vi "test-transform2d.vi"() -> ()   [LabVIEW 2019]
uses:
  <vilib>/Rock Robotics/WPI/ThirdParty/JAS_Junk/TrajLib/Translation_Equals.vi
  <vilib>/Rock Robotics/WPI/ThirdParty/JAS_Junk/TrajLib/Rotation_Equals.vi
  <vilib>/Rock Robotics/WPI/ThirdParty/JAS_Junk/TrajLib/Transform_Create_PosePose.vi
  <vilib>/Rock Robotics/WPI/ThirdParty/JAS_Junk/TrajLib/Pose_TransformBy.vi
  <vilib>/Rock Robotics/WPI/ThirdParty/JAS_Junk/TrajLib/Util_CalcDist.vi
  <vilib>/Rock Robotics/WPI/ThirdParty/JAS_Junk/TrajLib/Rotation_UnaryMinus.vi
  <vilib>/Rock Robotics/WPI/ThirdParty/JAS_Junk/TrajLib/Translation_RotateBy.vi
  <vilib>/Rock Robotics/WPI/ThirdParty/JAS_Junk/TrajLib/Translation_Minus.vi
  <vilib>/Rock Robotics/WPI/ThirdParty/JAS_Junk/TrajLib/Rotation_Minus.vi
  <vilib>/Rock Robotics/WPI/ThirdParty/JAS_Junk/TrajLib/Translation_Plus.vi
  <vilib>/Rock Robotics/WPI/ThirdParty/JAS_Junk/TrajLib/Rotation_Plus.vi
  <vilib>/Rock Robotics/WPI/ThirdParty/JAS_Junk/TrajLib/Rotation_RotateBy.vi
  <vilib>/Rock Robotics/WPI/ThirdParty/JAS_Junk/TrajLib/Rotation_CreateXY.vi
  <vilib>/Rock Robotics/WPI/ThirdParty/JAS_Junk/TrajLib/Trajectory_Library.lvlib
panel:
  out "T5 - ANG = 43 Deg":dbl
  out "T5 - Y2 = 4.4":dbl
  out "T5 - X2= -3.33":dbl
  out "T5 - Y = 4.4":dbl
  out "T5 - X = -3.33":dbl
  out "T4 -- Deg -- 0":dbl
  out "T4 -- y -- 0":dbl
  out "T4 -- X -- 0":dbl
  out "T3 - False":bool
  out "T2 - True":bool
  out "T1 -- Deg -- 0":dbl
  out "T1 -- y -- 0":dbl
  out "T1 -- X -- 0":dbl
  out "T0 -- Deg -- 0":dbl
  out "T0 -- y -- 0":dbl
  out "T0 -- X -- 0":dbl
  # "Transform2D Test  --- NOT DONE"
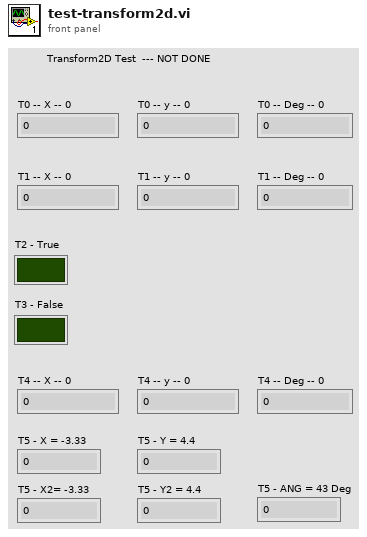
[diagram p1: front panel]
types:
  T1 = typedef "Trajectory_Library.lvlib/TRANSLATION2D.ctl" = cluster{"X":dbl, "Y":dbl}
  T2 = typedef "Trajectory_Library.lvlib/ROTATION2D.ctl" = cluster{"VALUE":dbl, "COS":dbl, "SIN":dbl}
  T3 = typedef "Trajectory_Library.lvlib/POSE2D.ctl" = cluster{"TRANSLATION":T1, "ROTATION":T2}
  T4 = typedef "Trajectory_Library.lvlib/TRANSFORM2D.ctl" = cluster{"TRANSLATION":T1, "ROTATION":T2}
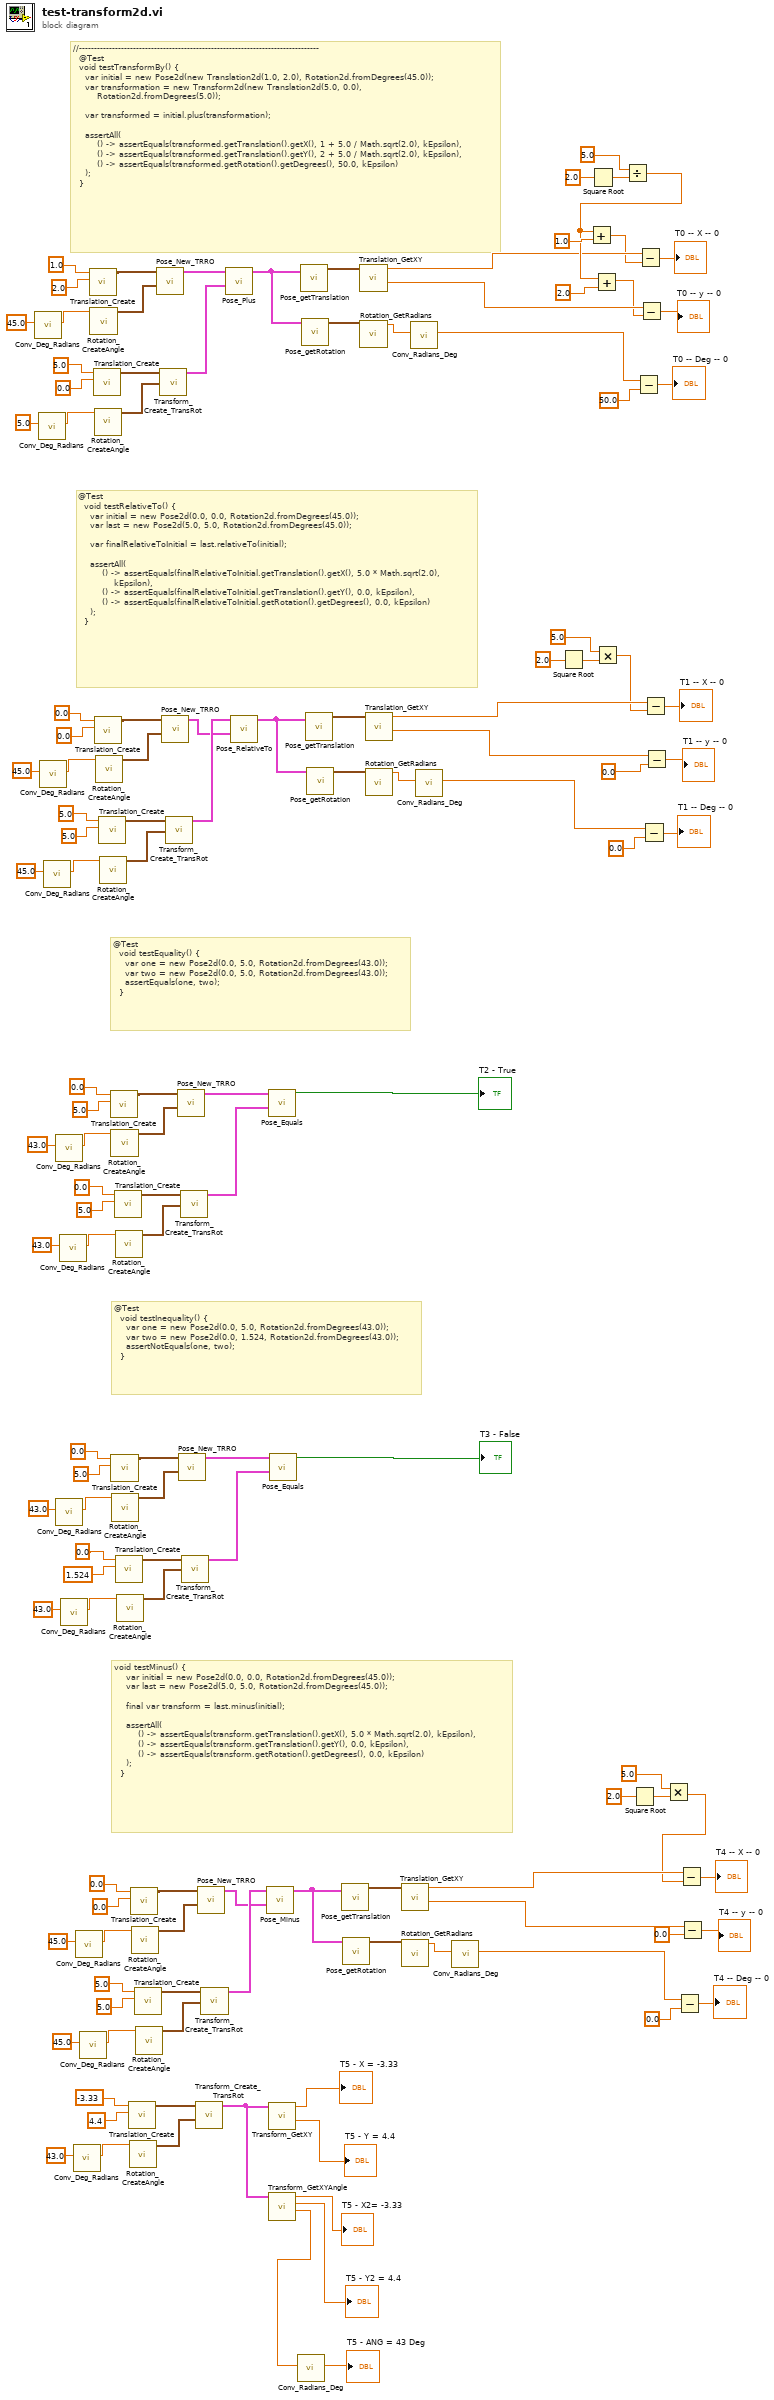
[diagram p0: block diagram]
diagram:
  # "void testMinus() {\n    var initial = new Pose2d(0.0, 0.0, Rotation2d.fromDegrees(45.0));\n    var last = new Pose2d(5.0, 5.0, Rotation2d.fromDegrees(45.0));\n\n    final var transform = last.minus(initial);\n\n    assertAll(\n        () -> assertEquals(transform.getTranslation().getX(), 5.0 * Math.sqrt(2.0), kEpsilon),\n        () -> assertEquals(transform.getTranslation().getY(), 0.0, kEpsilon),\n        () -> assertEquals(transform.getRotation().getDegrees(), 0.0, kEpsilon)\n    );\n  }"
  # "@Test\n  void testInequality() {\n    var one = new Pose2d(0.0, 5.0, Rotation2d.fromDegrees(43.0));\n    var two = new Pose2d(0.0, 1.524, Rotation2d.fromDegrees(43.0));\n    assertNotEquals(one, two);\n  }"
  # "@Test\n  void testEquality() {\n    var one = new Pose2d(0.0, 5.0, Rotation2d.fromDegrees(43.0));\n    var two = new Pose2d(0.0, 5.0, Rotation2d.fromDegrees(43.0));\n    assertEquals(one, two);\n  }"
  # "@Test\n  void testRelativeTo() {\n    var initial = new Pose2d(0.0, 0.0, Rotation2d.fromDegrees(45.0));\n    var last = new Pose2d(5.0, 5.0, Rotation2d.fromDegrees(45.0));\n\n    var finalRelativeToInitial = last.relativeTo(initial);\n\n    assertAll(\n        () -> assertEquals(finalRelativeToInitial.getTranslation().getX(), 5.0 * Math.sqrt(2.0),\n            kEpsilon),\n        () -> assertEquals(finalRelativeToInitial.getTranslation().getY(), 0.0, kEpsilon),\n        () -> assertEquals(finalRelativeToInitial.getRotation().getDegrees(), 0.0, kEpsilon)\n    );\n  }"
  # "//--------------------------------------------------------------------------------\n  @Test\n  void testTransformBy() {\n    var initial = new Pose2d(new Translation2d(1.0, 2.0), Rotation2d.fromDegrees(45.0));\n    var transformation = new Transform2d(new Translation2d(5.0, 0.0),\n        Rotation2d.fromDegrees(5.0));\n\n    var transformed = initial.plus(transformation);\n\n    assertAll(\n        () -> assertEquals(transformed.getTranslation().getX(), 1 + 5.0 / Math.sqrt(2.0), kEpsilon),\n        () -> assertEquals(transformed.getTranslation().getY(), 2 + 5.0 / Math.sqrt(2.0), kEpsilon),\n        () -> assertEquals(transformed.getRotation().getDegrees(), 50.0, kEpsilon)\n    );\n  }"
  n1 = call <vilib>:"Conv_Deg_Radians.vi"("Degress"=45.0) -> ("Radians"=w131:dbl)  [unwired: 10 in]
  n2 = call <vilib>:"Conv_Deg_Radians.vi"("Degress"=5.0) -> ("Radians"=w126:dbl)  [unwired: 10 in]
  n3 = call <vilib>:"Conv_Deg_Radians.vi"("Degress"=45.0) -> ("Radians"=w98:dbl)  [unwired: 10 in]
  n4 = call <vilib>:"Conv_Deg_Radians.vi"("Degress"=45.0) -> ("Radians"=w93:dbl)  [unwired: 10 in]
  n5 = call <vilib>:"Conv_Deg_Radians.vi"("Degress"=43.0) -> ("Radians"=w70:dbl)  [unwired: 10 in]
  n6 = call <vilib>:"Conv_Deg_Radians.vi"("Degress"=43.0) -> ("Radians"=w55:dbl)  [unwired: 10 in]
  n7 = call <vilib>:"Conv_Deg_Radians.vi"("Degress"=43.0) -> ("Radians"=w65:dbl)  [unwired: 10 in]
  n8 = call <vilib>:"Conv_Deg_Radians.vi"("Degress"=43.0) -> ("Radians"=w50:dbl)  [unwired: 10 in]
  n9 = call <vilib>:"Conv_Deg_Radians.vi"("Degress"=43.0) -> ("Radians"=w10:dbl)  [unwired: 10 in]
  n10 = call <vilib>:"Conv_Deg_Radians.vi"("Degress"=45.0) -> ("Radians"=w38:dbl)  [unwired: 10 in]
  n11 = call <vilib>:"Conv_Deg_Radians.vi"("Degress"=45.0) -> ("Radians"=w33:dbl)  [unwired: 10 in]
  n12 = call <vilib>:"Translation_Create.vi"("Y"=2.0, "X"=1.0) -> ("TRANSLATION"=w130:T1)  [unwired: 9 in]
  n13 = call <vilib>:"Rotation_CreateAngle.vi"("Angle"=w131) -> ("ROTATION"=w129:T2)  [unwired: 10 in]
  n14 = call <vilib>:"Translation_Create.vi"("Y"=0.0, "X"=5.0) -> ("TRANSLATION"=w124:T1)  [unwired: 9 in]
  n15 = call <vilib>:"Rotation_CreateAngle.vi"("Angle"=w126) -> ("ROTATION"=w123:T2)  [unwired: 10 in]
  n16 = call <vilib>:"Translation_Create.vi"("Y"=0.0, "X"=0.0) -> ("TRANSLATION"=w97:T1)  [unwired: 9 in]
  n17 = call <vilib>:"Rotation_CreateAngle.vi"("Angle"=w98) -> ("ROTATION"=w96:T2)  [unwired: 10 in]
  n18 = call <vilib>:"Translation_Create.vi"("Y"=5.0, "X"=5.0) -> ("TRANSLATION"=w91:T1)  [unwired: 9 in]
  n19 = call <vilib>:"Rotation_CreateAngle.vi"("Angle"=w93) -> ("ROTATION"=w90:T2)  [unwired: 10 in]
  n20 = call <vilib>:"Translation_Create.vi"("Y"=5.0, "X"=0.0) -> ("TRANSLATION"=w69:T1)  [unwired: 9 in]
  n21 = call <vilib>:"Rotation_CreateAngle.vi"("Angle"=w70) -> ("ROTATION"=w68:T2)  [unwired: 10 in]
  n22 = call <vilib>:"Translation_Create.vi"("Y"=5.0, "X"=0.0) -> ("TRANSLATION"=w54:T1)  [unwired: 9 in]
  n23 = call <vilib>:"Rotation_CreateAngle.vi"("Angle"=w55) -> ("ROTATION"=w53:T2)  [unwired: 10 in]
  n24 = call <vilib>:"Translation_Create.vi"("Y"=5.0, "X"=0.0) -> ("TRANSLATION"=w63:T1)  [unwired: 9 in]
  n25 = call <vilib>:"Rotation_CreateAngle.vi"("Angle"=w65) -> ("ROTATION"=w62:T2)  [unwired: 10 in]
  n26 = call <vilib>:"Translation_Create.vi"("Y"=1.524, "X"=0.0) -> ("TRANSLATION"=w48:T1)  [unwired: 9 in]
  n27 = call <vilib>:"Rotation_CreateAngle.vi"("Angle"=w50) -> ("ROTATION"=w47:T2)  [unwired: 10 in]
  n28 = call <vilib>:"Translation_Create.vi"("Y"=4.4, "X"=-3.33) -> ("TRANSLATION"=w9:T1)  [unwired: 9 in]
  n29 = call <vilib>:"Rotation_CreateAngle.vi"("Angle"=w10) -> ("ROTATION"=w8:T2)  [unwired: 10 in]
  n30 = call <vilib>:"Translation_Create.vi"("Y"=0.0, "X"=0.0) -> ("TRANSLATION"=w37:T1)  [unwired: 9 in]
  n31 = call <vilib>:"Rotation_CreateAngle.vi"("Angle"=w38) -> ("ROTATION"=w36:T2)  [unwired: 10 in]
  n32 = call <vilib>:"Translation_Create.vi"("Y"=5.0, "X"=5.0) -> ("TRANSLATION"=w31:T1)  [unwired: 9 in]
  n33 = call <vilib>:"Rotation_CreateAngle.vi"("Angle"=w33) -> ("ROTATION"=w30:T2)  [unwired: 10 in]
  n34 = call <vilib>:"Pose_New_TRRO.vi"("ROTATION"=w129, "TRANSLATION"=w130) -> ("outPOSE"=w122:T3)  [unwired: 9 in]
  n35 = call <vilib>:"Transform_Create_TransRot.vi"("ROTATION"=w123, "TRANSLATION"=w124) -> ("TRANSFORM"=w121:T4)  [unwired: 9 in]
  n36 = call <vilib>:"Pose_New_TRRO.vi"("ROTATION"=w96, "TRANSLATION"=w97) -> ("outPOSE"=w75:T3)  [unwired: 9 in]
  n37 = call <vilib>:"Transform_Create_TransRot.vi"("ROTATION"=w90, "TRANSLATION"=w91) -> ("TRANSFORM"=w76:T4)  [unwired: 9 in]
  n38 = call <vilib>:"Pose_New_TRRO.vi"("ROTATION"=w68, "TRANSLATION"=w69) -> ("outPOSE"=w61:T3)  [unwired: 9 in]
  n39 = call <vilib>:"Pose_New_TRRO.vi"("ROTATION"=w53, "TRANSLATION"=w54) -> ("outPOSE"=w46:T3)  [unwired: 9 in]
  n40 = call <vilib>:"Transform_Create_TransRot.vi"("ROTATION"=w62, "TRANSLATION"=w63) -> ("TRANSFORM"=w60:T4)  [unwired: 9 in]
  n41 = call <vilib>:"Transform_Create_TransRot.vi"("ROTATION"=w47, "TRANSLATION"=w48) -> ("TRANSFORM"=w45:T4)  [unwired: 9 in]
  n42 = call <vilib>:"Transform_Create_TransRot.vi"("ROTATION"=w8, "TRANSLATION"=w9) -> ("TRANSFORM"=w5:T4)  [unwired: 9 in]
  n43 = call <vilib>:"Pose_New_TRRO.vi"("ROTATION"=w36, "TRANSLATION"=w37) -> ("outPOSE"=w16:T3)  [unwired: 9 in]
  n44 = call <vilib>:"Transform_Create_TransRot.vi"("ROTATION"=w30, "TRANSLATION"=w31) -> ("TRANSFORM"=w17:T4)  [unwired: 9 in]
  n45 = call <vilib>:"Pose_Plus.vi"("other TRANSFORM"=w121, "in POSE"=w122) -> ("out POSE"=w119:T3)  [unwired: 9 in]
  n46 = call <vilib>:"Pose_RelativeTo.vi"("other POSE"=w75, "in POSE"=w76) -> ("out POSE"=w88:T3)  [unwired: 9 in]
  n47 = call <vilib>:"Pose_Minus.vi"("other TRANSFORM"=w16, "in POSE"=w17) -> ("outTRANSFORM"=w28:T4)  [unwired: 9 in]
  n48 = call <vilib>:"Pose_Equals.vi"("other POSE"=w60, "in POSE"=w61) -> ("Equals"=→"T2 - True":bool)  [unwired: 9 in]
  n49 = call <vilib>:"Transform_GetXY.vi"("inTRANSFORM"=w5) -> ("Y"=→"T5 - Y = 4.4":dbl, "X"=→"T5 - X = -3.33":dbl)  [unwired: 9 in]
  n50 = call <vilib>:"Transform_GetXYAngle.vi"("inTRANSFORM"=w5) -> ("Angle"=w1:dbl, "Y"=→"T5 - Y2 = 4.4":dbl, "X"=→"T5 - X2= -3.33":dbl)  [unwired: 8 in]
  n51 = call <vilib>:"Pose_Equals.vi"("other POSE"=w45, "in POSE"=w46) -> ("Equals"=→"T3 - False":bool)  [unwired: 9 in]
  n52 = call <vilib>:"Conv_Radians_Deg.vi"("Radians"=w1) -> ("Degrees"=→"T5 - ANG = 43 Deg":dbl)  [unwired: 10 in]
  n53 = call <vilib>:"Pose_getTranslation.vi"("in POSE"=w119) -> ("outTRANSLATION"=w120:T1)  [unwired: 10 in]
  n54 = call <vilib>:"Pose_getRotation.vi"("in POSE"=w119) -> ("out ROTATION"=w118:T2)  [unwired: 10 in]
  n55 = call <vilib>:"Pose_getTranslation.vi"("in POSE"=w88) -> ("outTRANSLATION"=w89:T1)  [unwired: 10 in]
  n56 = call <vilib>:"Pose_getRotation.vi"("in POSE"=w88) -> ("out ROTATION"=w87:T2)  [unwired: 10 in]
  n57 = call <vilib>:"Pose_getTranslation.vi"("in POSE"=w28) -> ("outTRANSLATION"=w29:T1)  [unwired: 10 in]
  n58 = call <vilib>:"Pose_getRotation.vi"("in POSE"=w28) -> ("out ROTATION"=w27:T2)  [unwired: 10 in]
  n59 = call <vilib>:"Translation_GetXY.vi"("In Translation"=w120) -> ("Y"=w108:dbl, "X"=w109:dbl)  [unwired: 9 in]
  n60 = call <vilib>:"Rotation_GetRadians.vi"("in ROTATION"=w118) -> ("AngleRadians"=w117:dbl)  [unwired: 10 in]
  n61 = call <vilib>:"Translation_GetXY.vi"("In Translation"=w89) -> ("Y"=w80:dbl, "X"=w81:dbl)  [unwired: 9 in]
  n62 = call <vilib>:"Rotation_GetRadians.vi"("in ROTATION"=w87) -> ("AngleRadians"=w86:dbl)  [unwired: 10 in]
  n63 = call <vilib>:"Translation_GetXY.vi"("In Translation"=w29) -> ("Y"=w20:dbl, "X"=w21:dbl)  [unwired: 9 in]
  n64 = call <vilib>:"Rotation_GetRadians.vi"("in ROTATION"=w27) -> ("AngleRadians"=w26:dbl)  [unwired: 10 in]
  n65 = call <vilib>:"Conv_Radians_Deg.vi"("Radians"=w117) -> ("Degrees"=w104:dbl)  [unwired: 10 in]
  n66 = call <vilib>:"Conv_Radians_Deg.vi"("Radians"=w86) -> ("Degrees"=w78:dbl)  [unwired: 10 in]
  n67 = call <vilib>:"Conv_Radians_Deg.vi"("Radians"=w26) -> ("Degrees"=w18:dbl)  [unwired: 10 in]
  n68 = Square Root(x=2.0) -> (sqrt(x)=w84:dbl)
  n69 = Square Root(x=2.0) -> (sqrt(x)=w115:dbl)
  n70 = Multiply(x=5.0, y=w84) -> (x*y=w74:dbl)
  n71 = Divide(x=5.0, y=w115) -> (x/y=w111:dbl)
  n72 = Add(x=w111, y=1.0) -> (x+y=w106:dbl)
  n73 = Add(x=w111, y=2.0) -> (x+y=w107:dbl)
  n74 = Square Root(x=2.0) -> (sqrt(x)=w24:dbl)
  n75 = Subtract(x=w104, y=50.0) -> (x-y=→"T0 -- Deg -- 0":dbl)
  n76 = Subtract(x=w109, y=w106) -> (x-y=→"T0 -- X -- 0":dbl)
  n77 = Subtract(x=w108, y=w107) -> (x-y=→"T0 -- y -- 0":dbl)
  n78 = Subtract(x=w78, y=0.0) -> (x-y=→"T1 -- Deg -- 0":dbl)
  n79 = Subtract(x=w81, y=w74) -> (x-y=→"T1 -- X -- 0":dbl)
  n80 = Subtract(x=w80, y=0.0) -> (x-y=→"T1 -- y -- 0":dbl)
  n81 = Multiply(x=5.0, y=w24) -> (x*y=w15:dbl)
  n82 = Subtract(x=w18, y=0.0) -> (x-y=→"T4 -- Deg -- 0":dbl)
  n83 = Subtract(x=w21, y=w15) -> (x-y=→"T4 -- X -- 0":dbl)
  n84 = Subtract(x=w20, y=0.0) -> (x-y=→"T4 -- y -- 0":dbl)
